vi "Main Page.vi"(8 "error in (no error)":errorcluster, 11 "Node Ptr":T1 format="%.0x") -> (0 "error out":errorcluster)   [LabVIEW 2015, in "SLSC Module Template System Explorer.lvlib"]
uses:
  SLSC Module Template System Explorer.lvlib
  <vilib>/NI Veristand/Custom Device API/Custom Device Item Ref.ctl
  Shared/Constants.vi
  <vilib>/NI Veristand/Custom Device API/Get Item Property (I32).vi
  <vilib>/NI Veristand/Custom Device API/Get Item Property (Variant).vi
  <vilib>/NI Veristand/Custom Device API/Set Item Property (Variant).vi
  <vilib>/NI Veristand/Custom Device API/Custom Device API.lvlib
  Shared/SLSC Module Template Shared.lvlib
panel:
  in  "*Bool..NI.GreenLED2":bool caption="LED2 Green"
  in  "Header 2":cluster{"Section Name":string}={"Section Name"="Custom Device Item Settings"}
  in  "*Bool.LED0.NI.RedBool":bool caption="LED0 Red"
  out "Debug Control":variant
  in  "*Bool.LED0.NI.GreenBool":bool caption="LED0 Green"
  out "Module Number":i32
  in  "Header":cluster{"Section Name":string}={"Section Name"="Custom Device Item Settings"}
  in  "Description":string
  in  "Name":string
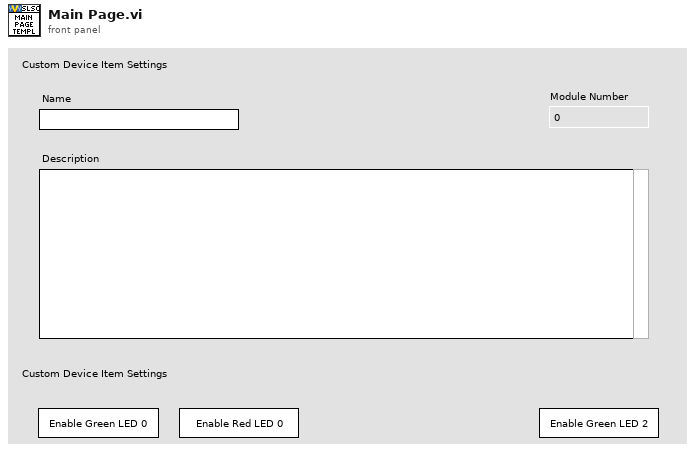
[diagram p1: front panel]
types:
  T1 = typedef "Custom Device API.lvlib/Custom Device Item Ref.ctl" = u64
  T2 = enum8{"Enabled", "Disabled", "Disabled and Grayed Out"}
  T3 = typedef "Custom Device API.lvlib/Custom Device Item Info.ctl" = cluster{"Name":string, "Is Channel":bool, "GUID":string, "Is Waveform":bool}
  T4 = typedef "Custom Device API.lvlib/Custom Device Commands.ctl" = enum16{"Default", "Item renamed", "Shutdown", "Dynamic button pressed"}
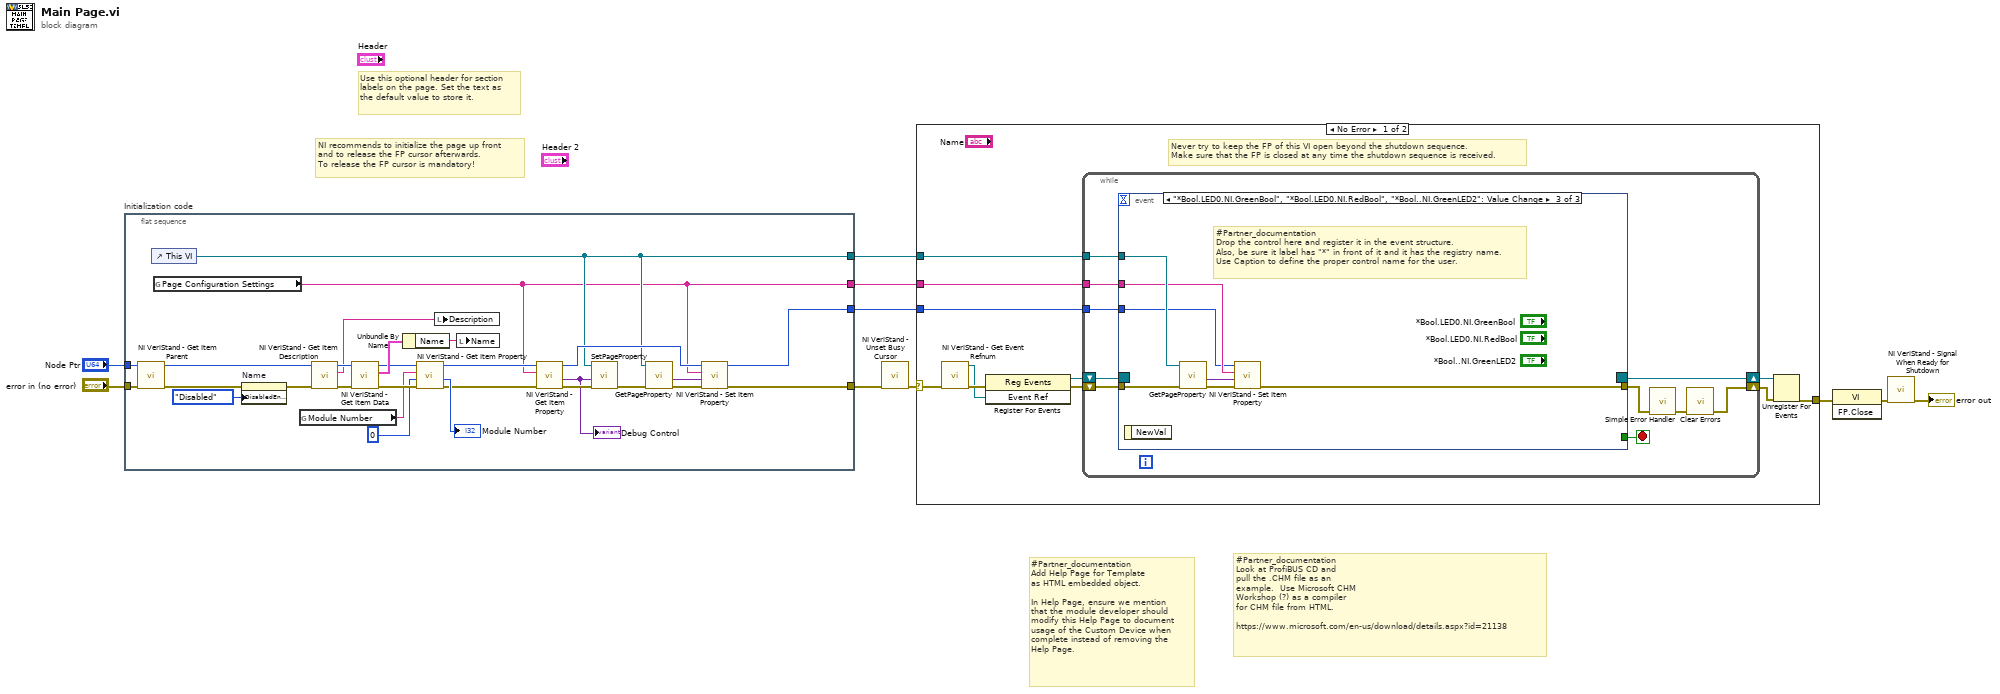
[diagram p0: block diagram]
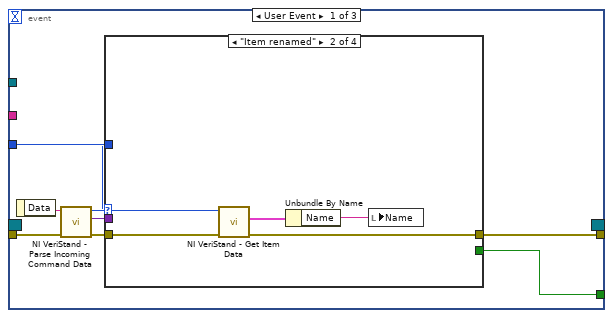
[diagram p2: hidden frame]
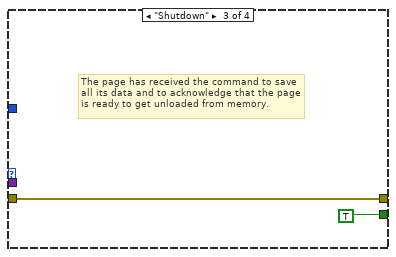
[diagram p4: hidden frame]
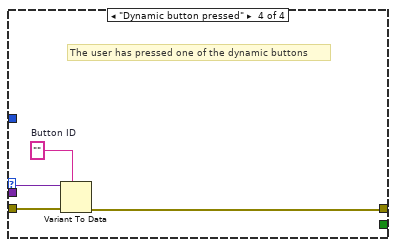
[diagram p5: hidden frame]
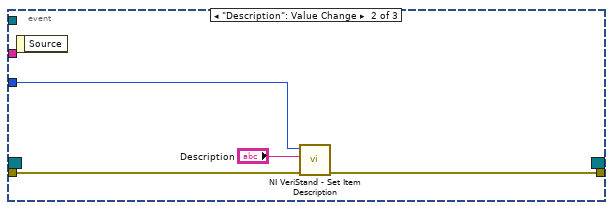
[diagram p6: hidden frame]
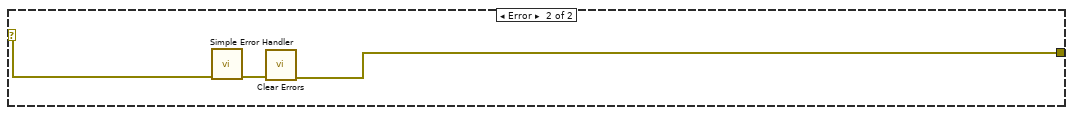
[diagram p7: hidden frame]
diagram:
  # "#Partner_documentation\nLook at ProfiBUS CD and\npull the .CHM file as an \nexample.  Use Microsoft CHM\nWorkshop (?) as a compiler\nfor CHM file from HTML.\n\nhttps://www.microsoft.com/en-us/download/details.aspx?id=21138"
  # "#Partner_documentation\nAdd Help Page for Template\nas HTML embedded object.\n\nIn Help Page, ensure we mention\nthat the module developer should\nmodify this Help Page to document\nusage of the Custom Device when\ncomplete instead of removing the \nHelp Page."
  # "Use this optional header for section labels on the page. Set the text as the default value to store it."
  # "NI recommends to initialize the page up front\nand to release the FP cursor afterwards.\nTo release the FP cursor is mandatory!"
  n1 = flat-sequence "Initialization code" {
    tunnel: "error in (no error)" -> [w13]
    tunnel: "Node Ptr" -> [w14]
    tunnel: [w20] -> w6
    tunnel: [w17] -> w3
    tunnel: [w16] -> w2
    tunnel: [w15] -> w1
    frame #0 {
      n2 = call <vilib>:"NI VeriStand - Get Item Parent.vi"("error in (no error)"=w13, "Item Ref in"=w14) -> ("error out"=w11:errorcluster, "Item Ref out"=w12:T1)  [unwired: 6 in, 2 out]
      n3 = control-ref of="This VI"() -> (w16:refnum<vi>)
      n4 = global read "Constants.vi" "Page Configuration Settings"() -> (w15:string)
      n5 = property on="Name" class="Str"(error in=w11, "DisabledEnum"=T2."Disabled" ("Disabled")) -> (error out=w32:errorcluster)  [unwired: 1 in, 1 out]
      n6 = global read "Constants.vi" "Module Number"() -> (w29:string)
      n7 = call <vilib>:"NI VeriStand - Get Item Description.vi"("error in (no error)"=w32, "Item Ref in"=w12) -> ("error out"=w36:errorcluster, "Description"=w37:string, "Item Ref out"=w38:T1)  [unwired: 7 out]
      n8 = call <vilib>:"NI VeriStand - Get Item Data.vi"("error in (no error)"=w36, "Item Ref in"=w38) -> ("error out"=w30:errorcluster, "Item Info"=w35:T3, "Item Ref out"=w28:T1)  [unwired: 7 out]
      n9 = Unbundle By Name(w35) -> ("Name"=w34:string)
      n10 = call-poly <vilib>:"NI VeriStand - Get Item Property.vi"("error in (no error)"=w30, "Default Value"=0, "Property Name"=w29, "Item Ref in"=w28) -> ("error out"=w25:errorcluster, "Value"=→"Module Number":i32, "Item Ref out"=w26:T1)  [unwired: 4 in, 1 out]
      n11 = local write "Description"(w37) -> ()
      n12 = local write "Name"(w34) -> ()
      n13 = call-poly <vilib>:"NI VeriStand - Get Item Property.vi"("error in (no error)"=w25, "Property Name"=w15, "Item Ref in"=w26) -> ("error out"=w24:errorcluster, "Value"=w23:variant, "Item Ref out"=w19:T1)  [unwired: 5 in, 1 out]
      "Debug Control" <- w23
      n14 = call "SetPageProperty.vi"("error in"=w24, "variant"=w23, "This VI"=w16) -> ("error out"=w22:errorcluster)  [unwired: 8 in]
      n15 = call "GetPageProperty.vi"("error in (no error)"=w22, "This VI"=w16) -> ("error out"=w21:errorcluster, "Settings"=w18:variant)  [unwired: 8 in]
      n16 = call-poly <vilib>:"NI VeriStand - Set Item Property.vi"("error in (no error)"=w21, "Value"=w18, "Property Name"=w15, "Item Ref in"=w19) -> ("error out"=w20:errorcluster, "Item Ref out"=w17:T1)  [unwired: 5 in, 1 out]
    }
  }
  n17 = call <vilib>:"NI VeriStand - Unset Busy Cursor.vi"("error in (no error)"=w6) -> ("error out"=w5:errorcluster)  [unwired: 10 out]
  n18 = case shown="No Error" w5 {
    selector: w5 -> [w41 w93]
    tunnel: [w46 w91] -> w10
    tunnel: w3 -> [w42 _]
    tunnel: w2 -> [w40 _]
    tunnel: w1 -> [w39 _]
    frame No Error {
      # "Never try to keep the FP of this VI open beyond the shutdown sequence.\nMake sure that the FP is closed at any time the shutdown sequence is received."
      n19 = call <vilib>:"NI VeriStand - Get Event Refnum.vi"("error in (no error)"=w41) -> ("error out"=w49:errorcluster, "Event Ref"=w45:refnum<user-event>)  [unwired: 9 out]
      n20 = register-events(error in=w49, w45) -> (reference out=w43:refnum<event-registration>, error out=w44:errorcluster)  [unwired: 1 in]
      n21 = while {
        tunnel: w42 -> [w55]
        shift-right: [w52] -> w47
        shift-left: w44 -> [w58]
        shift-right: [w59] -> w48
        shift-left: w43 -> [w57]
        tunnel: w40 -> [w51]
        tunnel: w39 -> [w50]
        stop <- w56 stop-if-true
        n22 = event shown="[2] \"*Bool.LED0.NI.GreenBool\", \"*Bool.LED0.NI.RedBool\", \"*Bool..NI.GreenLED2\": Value Change" {
          selector: w57 -> [_ _ _]
          dyn-events: [_ _ _] -> w59
          timeout: _ -> [_ _ _]
          tunnel: w58 -> [w67 w82 w90]
          tunnel: [w63 _ _] -> w56
          tunnel: [w62 w81 w87] -> w54
          tunnel: w55 -> [w61 w83 w84]
          tunnel: w51 -> [_ _ w89]
          tunnel: w50 -> [_ _ w86]
          event User Event {
            n23 = event-data() -> ("Data"=w66:string)  [unwired: 1 out]
            n24 = call <vilib>:"NI VeriStand - Parse Incoming Command Data.vi"("error in (no error)"=w67, "Incoming data"=w66) -> ("error out"=w65:errorcluster, "Outgoing data"=w60:variant, "Action"=w64:T4)  [unwired: 7 out]
            n25 = case shown="\"Item renamed\"" w64 {
              tunnel: w65 -> [w68 w73 w74 w79]
              tunnel: [_ _ TRUE _] -> w63
              tunnel: [w68 w70 w74 w76] -> w62
              tunnel: w61 -> [_ w72 _ _]
              tunnel: w60 -> [_ _ _ w78]
              frame "Default", Default {
              }
              frame "Item renamed" {
                n26 = call <vilib>:"NI VeriStand - Get Item Data.vi"("error in (no error)"=w73, "Item Ref in"=w72) -> ("error out"=w70:errorcluster, "Item Info"=w71:T3)  [unwired: 8 out]
                n27 = Unbundle By Name(w71) -> ("Name"=w69:string)
                n28 = local write "Name"(w69) -> ()
              }
              frame "Shutdown" {
                # "The page has received the command to save all its data and to acknowledge that the page is ready to get unloaded from memory."
              }
              frame "Dynamic button pressed" {
                w77 = ""  # Button ID
                # "The user has pressed one of the dynamic buttons"
                n29 = Variant To Data(error in=w79, type=w77, Variant=w78) -> (error out=w76:errorcluster)  [unwired: 1 out]
              }
            }
          }
          event "Description": Value Change {
            n30 = event-data() -> ()  [unwired: 2 out]
            n31 = call <vilib>:"NI VeriStand - Set Item Description.vi"("error in (no error)"=w82, "Description"="Description", "Item Ref in"=w83) -> ("error out"=w81:errorcluster)  [unwired: 8 out]
          }
          event "*Bool.LED0.NI.GreenBool", "*Bool.LED0.NI.RedBool", "*Bool..NI.GreenLED2": Value Change {
            # "#Partner_documentation\nDrop the control here and register it in the event structure.\nAlso, be sure it label has \"*\" in front of it and it has the registry name.\nUse Caption to define the proper control name for the user."
            n32 = event-data() -> ()  [unwired: 2 out]
            n33 = call "GetPageProperty.vi"("error in (no error)"=w90, "This VI"=w89) -> ("error out"=w88:errorcluster, "Settings"=w85:variant)  [unwired: 8 in]
            n34 = call-poly <vilib>:"NI VeriStand - Set Item Property.vi"("error in (no error)"=w88, "Value"=w85, "Property Name"=w86, "Item Ref in"=w84) -> ("error out"=w87:errorcluster)  [unwired: 5 in, 2 out]
          }
        }
        n35 = call <vilib>:"Simple Error Handler.vi"("error in (no error)"=w54) -> ("error out"=w53:errorcluster)  [unwired: 1 in, 7 out]
        n36 = call <vilib>:"Clear Errors.vi"("error in (no error)"=w53) -> ("error out"=w52:errorcluster)  [unwired: 1 in, 5 out]
      }
      n37 = Unregister For Events(event registration refnum=w48, error in=w47) -> (error out=w46:errorcluster)
    }
    frame Error {
      n38 = call <vilib>:"Simple Error Handler.vi"("error in (no error)"=w93) -> ("error out"=w92:errorcluster)  [unwired: 1 in, 7 out]
      n39 = call <vilib>:"Clear Errors.vi"("error in (no error)"=w92) -> ("error out"=w91:errorcluster)  [unwired: 1 in, 5 out]
    }
  }
  n40 = invoke class="VI" method="FP.Close"(error in=w10) -> (error out=w9:errorcluster)  [unwired: 2 in, 2 out]
  n41 = call <vilib>:"NI VeriStand - Signal When Ready for Shutdown.vi"("error in (no error)"=w9) -> ("error out"=→"error out":errorcluster)  [unwired: 10 out]
